vi "Write timedelays.vi"(8 "error in (no error)":errorcluster, 10 "timedelays":dbl[](array[numeric]), 11 "DATA in":refnum<class "DATA.lvclass">) -> (0 "error out":errorcluster, 3 "DATA out":refnum<class "DATA.lvclass">)   [LabVIEW 2020, in "DATA.lvclass"]
uses:
  DATA.lvclass
  DATA.lvclass/DATA.ctl
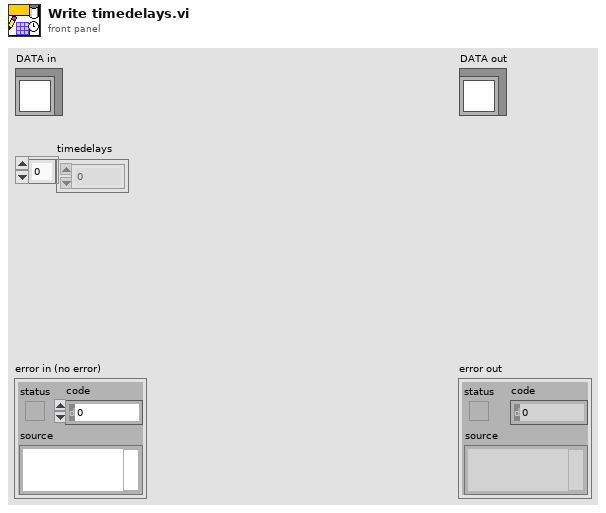
[diagram p1: front panel]
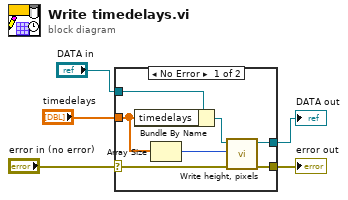
[diagram p0: block diagram]
diagram:
  n1 = case shown="No Error" "error in (no error)" {
    selector: "error in (no error)" -> [w12 w13]
    tunnel: [w11 w13] -> w4
    tunnel: [w9 w14] -> w2
    tunnel: "DATA in" -> [w8 w14]
    tunnel: "timedelays" -> [w7 _]
    frame No Error {
      n2 = Bundle By Name(cluster=w8, "timedelays"=w7) -> (w10:refnum<class "DATA.lvclass">)
      n3 = Array Size(array=w7) -> (size(s)=w6:i32)
      n4 = call "Write height, pixels.vi"("error in (no error)"=w12, "height, pixels"=w6, "DATA in"=w10) -> ("error out"=w11:errorcluster, "DATA out"=w9:refnum<class "DATA.lvclass">)  [unwired: 7 in]
    }
    frame Error {
    }
  }
  "error out" <- w4
  "DATA out" <- w2
